vi "DataWrapper.vi"(6 "Destination":string, 7 "Source":string, 8 "error in (no error)":errorcluster, 9 "value":variant, 10 "Description":string, 11 "GRMActor in":refnum<class "GeneralRMActor.lvclass">) -> (0 "error out":errorcluster, 2 "DataExchange":T1, 3 "GRMActor out":refnum<class "GeneralRMActor.lvclass">)   [LabVIEW 2020, in "GeneralRMActor.lvlib" / "GeneralRMActor.lvclass"]
uses:
  GeneralRMActor.lvclass
  Device/Device/DataExchange.ctl
  Interface/DataListener/DataListener.lvclass
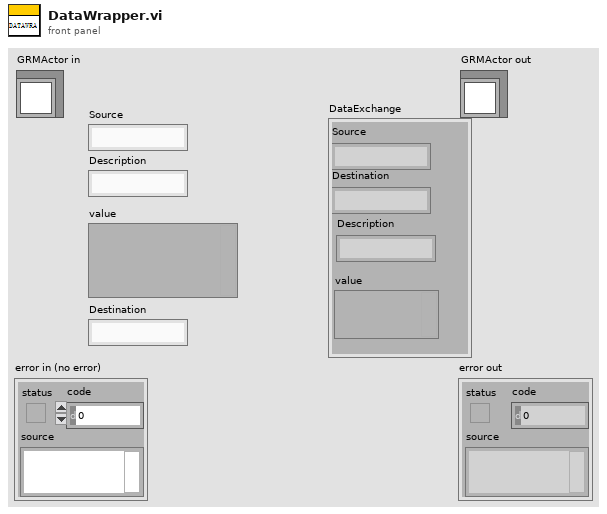
[diagram p1: front panel]
types:
  T1 = typedef "DataListener.lvclass/DataExchange.ctl" = cluster{"Source":string, "Destination":string, "Description":string, "value":variant}
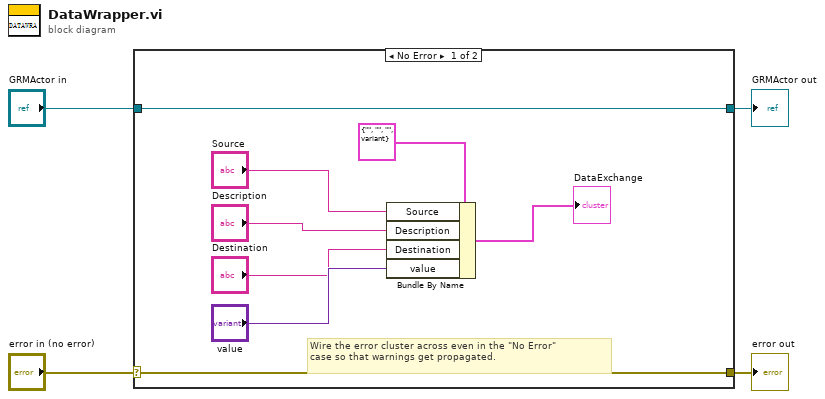
[diagram p0: block diagram]
diagram:
  n1 = case shown="No Error" "error in (no error)" {
    selector: "error in (no error)" -> [w11 w14]
    tunnel: [w11 w14] -> w3
    tunnel: [w12 w13] -> w1
    tunnel: "GRMActor in" -> [w12 w13]
    frame No Error {
      # "Wire the error cluster across even in the \"No Error\"\ncase so that warnings get propagated."
      n2 = Bundle By Name(cluster=T1 {"Source"="", "Destination"="", "Description"="", "value"=variant} ("DataExchange"), "Source"="Source", "Description"="Description", "Destination"="Destination", "value"="value") -> (→"DataExchange":T1)
    }
    frame Error {
    }
  }
  "error out" <- w3
  "GRMActor out" <- w1
